vi "TEST-PI.vi"() -> ()   [LabVIEW 2014]
panel:
  out "Names":string[](array[string])
  out "DRR? string":string
  out "Waveform Graph":dbl[][](graph)
  out "result":bool
  out "appended array":dbl[][](array[numeric])
  in  "N":i32=100
  in  "Nmax":i32=1024
  in  "System no.":i32=1 min=1 max=4 step=1
  in  "Axis":string
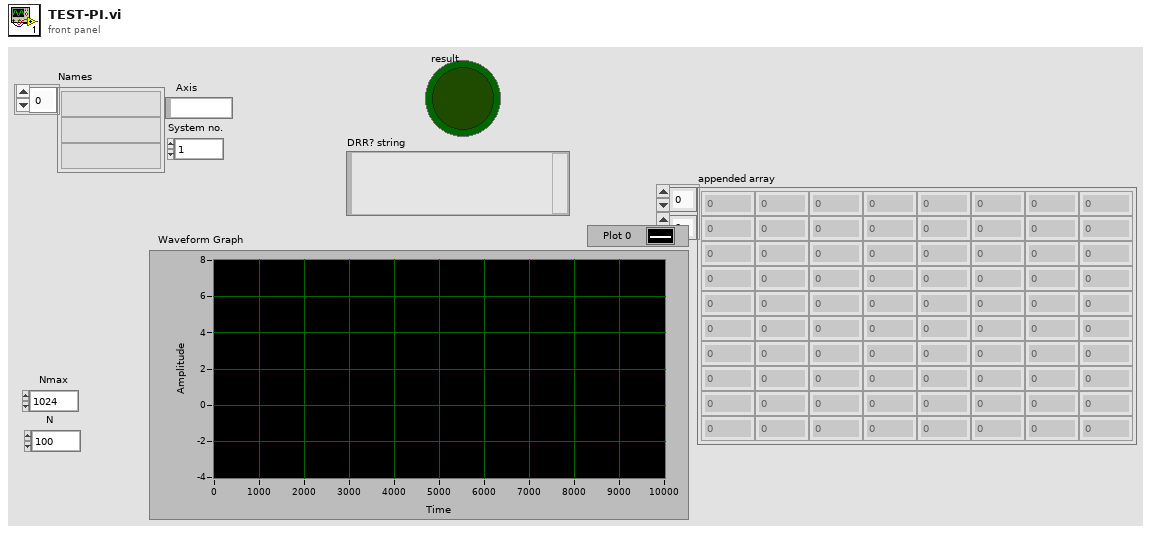
[diagram p1: front panel]
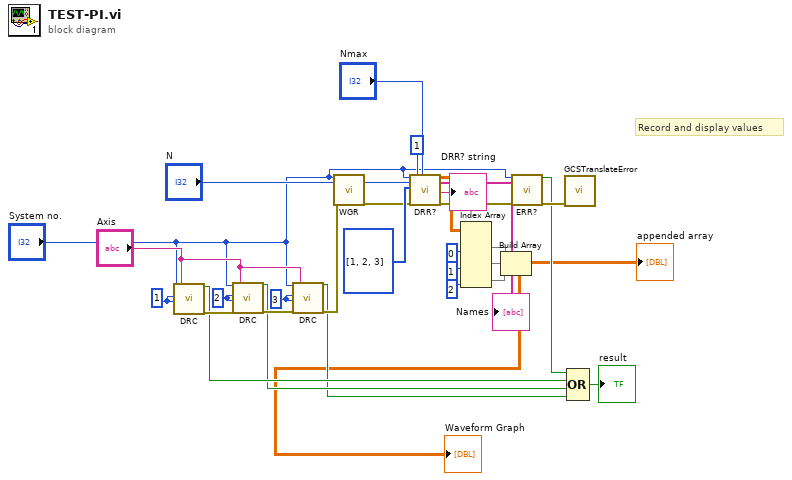
[diagram p0: block diagram]
diagram:
  w17 = 3 ("Numeric")
  w18 = 2 ("Numeric")
  w25 = 1 ("Numeric")
  # "Record and display values"
  n1 = call "DRC.vi"("System no."="System no.", "Rec. table"=w25, "Rec. option"=w25, "Source ID"="Axis") -> ("Controller error"=w15:bool, "error out"=w24:errorcluster)  [unwired: 2 in, 12 out]
  n2 = call "DRC.vi"("System no."="System no.", "Rec. table"=w18, "Rec. option"=w18, "error in"=w24, "Source ID"="Axis") -> ("Controller error"=w14:bool, "error out"=w23:errorcluster)  [unwired: 1 in, 12 out]
  n3 = call "DRC.vi"("System no."="System no.", "Rec. table"=w17, "Rec. option"=w17, "error in"=w23, "Source ID"="Axis") -> ("Controller error"=w13:bool, "error out"=w16:errorcluster)  [unwired: 1 in, 12 out]
  n4 = call "WGR.vi"("System no."="System no.", "error in"=w16) -> ("error out"=w11:errorcluster)  [unwired: 2 in, 15 out]
  n5 = call "DRR?.vi"("System no."="System no.", "Rec. table IDs"=i32[] [1, 2, 3], "error in"=w11, "Xo"=1, "N"="N", "Nmax"="Nmax") -> ("Data"=w28:dbl[][], "Names"=→"Names":string[], "DRR? string"=→"DRR? string":string, "error out"=w9:errorcluster)  [unwired: 2 in, 8 out]
  n6 = Index Array(array=w28, index (col) #1=0 ("Disabled Index (col)"), index (col) #2=1 ("Disabled Index (col)"), index (col) #3=2 ("Disabled Index (col)")) -> (element #1=w26:dbl[], element #2=w20:dbl[], element #3=w19:dbl[])  [unwired: 3 in]
  n7 = Build Array(w26, w20, w19) -> (→"appended array" →"Waveform Graph":dbl[][])
  n8 = call "ERR?.vi"("System no."="System no.", "error in"=w9) -> ("Controller error"=w10:bool, "error out"=w30:errorcluster)  [unwired: 16 out]
  n9 = call "GCSTranslateError.vi"("error in"=w30) -> ()  [unwired: 19 out]
  n10 = Compound Arithmetic op=OR(w10, w15, w14, w13) -> (→"result":bool)
